vi "BuildFullTag.vi"(10 "Cluster":T1, 11 "byte order":T2(ring)) -> (3 "String Out":string)   [LabVIEW 2022 SP3]
uses:
  miDataType.ctl
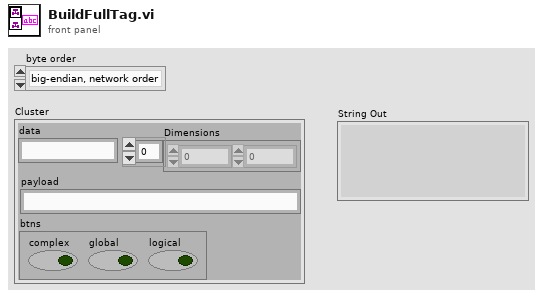
[diagram p1: front panel]
types:
  T1 = cluster{"data":string, "Dimensions":i32[], "payload":string, "btns":cluster{"complex":bool, "global":bool, "logical":bool}}
  T2 = enum16{"big-endian, network order", "native, host order", "little-endian"}
  T3 = typedef "miDataType.ctl" = enum16{"illegal", "miINT8", "miUINT8", "miINT16", "miUINT16", "miINT32", "miUINT32", "miSINGLE", "--", "miDOUBLE", "---", "----", "miINT64", "miUINT64", "miMATRIX", "miCOMPRESSED", "miUTF8", "miUTF16", "miUTF32", "udefined"}
  T4 = cluster{"Data Type":T3, "# bytes":u32, "data":string}
  T5 = enum16{"illegal", "Cell array", "Structure", "Object", "Character Array", "Sparse Array", "Double Array", "Single Array", "i8", "u8", "i16", "u16", "i32", "u32", "i64", "u64"}
  T6 = cluster{"complex":bool, "global":bool, "logical":bool}
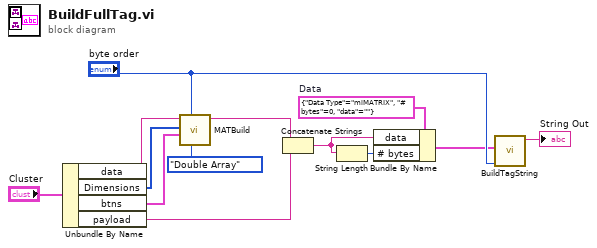
[diagram p0: block diagram]
diagram:
  w4 = T4 {"Data Type"=enum."miMATRIX", "# bytes"=0, "data"=""}  # Data
  n1 = Unbundle By Name("Cluster") -> ("data"=w10:string, "Dimensions"=w11:i32[], "btns"=w13:T6, "payload"=w1:string)
  n2 = call "MATBuild.vi"("Class in"=T5."Double Array" ("Class"), "byte order"="byte order", "Cluster"=w13, "Dimensions"=w11, "Name"=w10) -> ("String Out"=w7:string)  [unwired: 6 in]
  n3 = Concatenate Strings(w7, w1) -> (w5:string)
  n4 = String Length(string=w5) -> (length=w6:i32)
  n5 = Bundle By Name(cluster=w4, "data"=w5, "# bytes"=w6) -> (w3:T4)
  n6 = call "BuildTagString.vi"("byte order"="byte order", "Tag"=w3) -> ("String Out"=→"String Out":string)  [unwired: 8 in, 1 out]
